vi "open.vi"(8 "error in":errorcluster, 11 "IP Address":string="192.168.0.28") -> (0 "error out":errorcluster, 3 "MB_TCP session out":refnum<class "MB_Master_TCP.lvclass">)   [LabVIEW 2025, in "TanksPlcDriver.lvlib"]
uses:
  <vilib>/Plasmionique/MB Master/MB_Master_TCP/MB_Master_TCP.lvclass
  TanksPlcDriver.lvlib
panel:
  # "IO-Link  Driver V0.10\nOpen"
  # "09.04.2025"
  # "Andrej Valand"
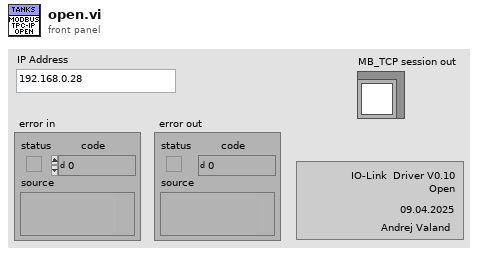
[diagram p1: front panel]
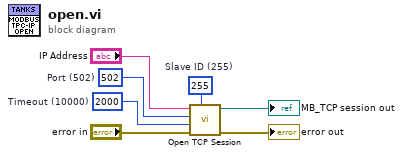
[diagram p0: block diagram]
diagram:
  w6 = u8 255  # Slave ID (255)
  w5 = u16 502  # Port (502)
  w4 = 2000  # Timeout (10000)
  n1 = call <vilib>:"Open TCP Session.vi"("Slave ID (255)"=w6, "error in (no error)"="error in", "Timeout (10000)"=w4, "Port (502)"=w5, "IP Address"="IP Address") -> ("error out"=→"error out":errorcluster, "MB_TCP session"=→"MB_TCP session out":refnum<class "MB_Master_TCP.lvclass">)  [unwired: 5 in]
